vi "Load Image From Binary File LV2012 NIVerified.vi"() -> ()   [LabVIEW 2018]
doc: "This VI demonstrates how to load an image saved as binary file and convert the data back into a LabVIEW picture."
panel:
  out "Pixels loaded":i32
  in  "Picture height":i32=283
  in  "Picture width":i32=305
  out "2D Picture":picture
  # "Overview: Demonstrates how to load an image saved as binary file and convert the data back into a LabVIEW picture.\nRequirements: LabVIEW Base Development System 2012 (or compatible)\nInstructions: \n1. Run the VI.\n2. Select BinaryImage.bin as file to load. This file can be created with Save Image As Binary File.vi."
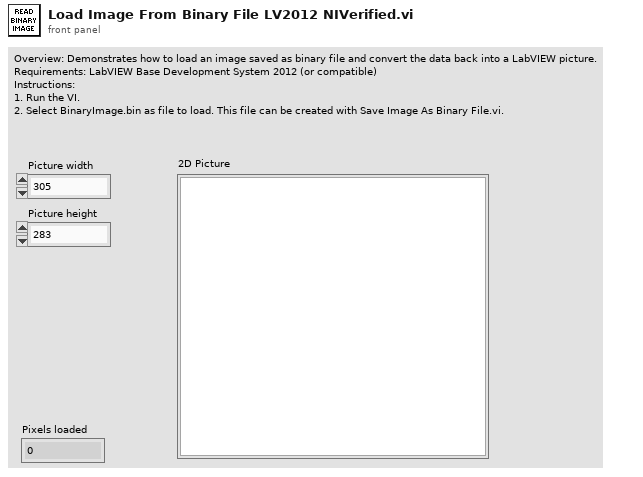
[diagram p1: front panel]
types:
  T1 = enum16{"big-endian, network order", "native, host order", "little-endian"}
  T2 = typedef "imagedata.ctl" = cluster{"image type":i32, "image depth":i32, "image":u8[], "mask":u8[], "colors":u32[], "Rectangle":cluster{"left":i16, "top":i16, "right":i16, "bottom":i16}}
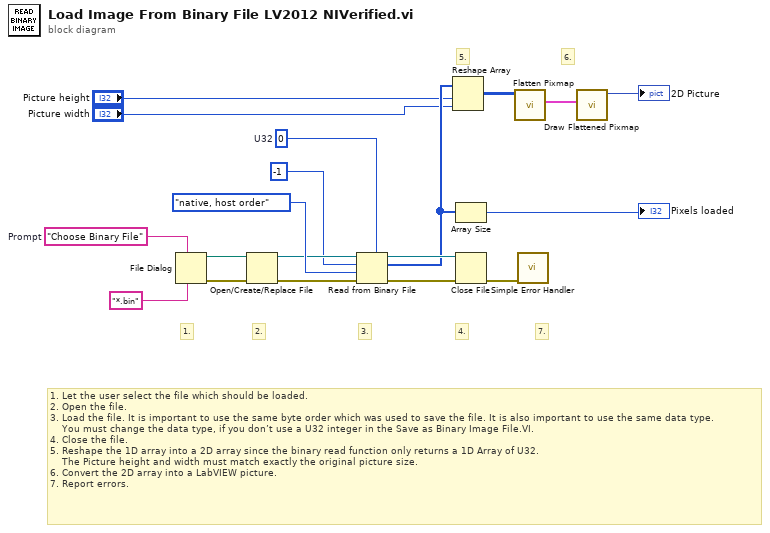
[diagram p0: block diagram]
diagram:
  w10 = u32 0  # U32
  w17 = "Choose Binary File"  # Prompt
  # "1. Let the user select the file which should be loaded.\n2. Open the file.\n3. Load the file. It is important to use the same byte order which was used to save the file. It is also important to use the same data type.\n    You must change the data type, if you don’t use a U32 integer in the Save as Binary Image File.VI.\n4. Close the file.\n5. Reshape the 1D array into a 2D array since the binary read function only returns a 1D Array of U32.\n    The Picture height and width must match exactly the original picture size.\n6. Convert the 2D array into a LabVIEW picture.\n7. Report errors."
  # "7."
  # "6."
  # "5."
  # "4."
  # "3."
  # "2."
  # "1."
  n1 = File Dialog(6:"*.bin" ("pattern (all files)"), 7:w17) -> (0:w15:errorcluster, 3:w18:path)  [unwired: 5 in, 2 out]
  n2 = Open/Create/Replace File(file path (use dialog)=w18, error in=w15) -> (refnum out=w11:refnum<file>, error out=w12:errorcluster)  [unwired: 4 in, 1 out]
  n3 = Read from Binary File(5:w10, 8:w12, 9:T1."native, host order" ("byte order (0:big-endian, network order)"), 10:-1 ("count (1)"), 11:w11) -> (0:w16:errorcluster, 2:w6:u32[], 3:w19:refnum<file>)  [unwired: 1 in, 1 out]
  n4 = Reshape Array(w6, "Picture height", "Picture width") -> (w1:u32[][])
  n5 = Array Size(array=w6) -> (size(s)=→"Pixels loaded":i32)
  n6 = Close File(refnum=w19, error in=w16) -> (error out=w5:errorcluster)  [unwired: 1 out]
  n7 = call <vilib>:"Flatten Pixmap.vi"("24-bit pixmap"=w1) -> ("image data"=w8:T2)  [unwired: 10 in]
  n8 = call <vilib>:"Simple Error Handler.vi"("error in (no error)"=w5) -> ()  [unwired: 4 in, 5 out]
  n9 = call <vilib>:"Draw Flattened Pixmap.vi"("image data"=w8) -> ("new picture"=→"2D Picture":picture)  [unwired: 8 in]
